vi "FGV Map Get Data (Variant).vi"(8 "error in (no error)":errorcluster, 10 "Data Key":string, 11 "Instance Key":string) -> (0 "error out":errorcluster, 2 "Data Not Found ?":bool, 3 "Data Out":variant)   [LabVIEW 2020, in "FGV Map.lvlib"]
uses:
  FGV Map.lvlib
  Controls/FGV Map Core State.ctl
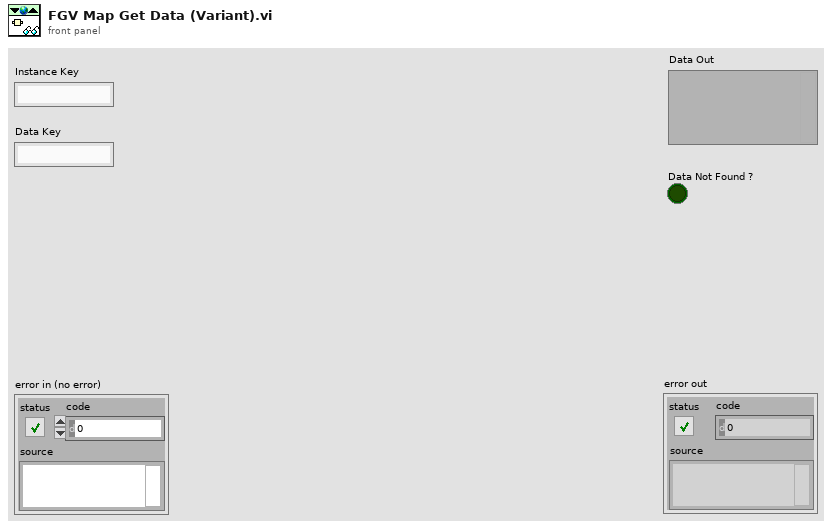
[diagram p1: front panel]
types:
  T1 = typedef "FGV Map.lvlib/FGV Map Core State.ctl" = enum16{"Init", "Set Instance (Unlock)", "Get Instance", "Get Instance (Lock)", "Unlock", "Get All Instances", "Delete Instance"}
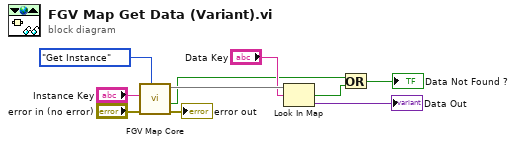
[diagram p0: block diagram]
diagram:
  n1 = call "FGV Map Core.vi"("FGV State"=FGV_Map_Core_State."Get Instance", "error in"="error in (no error)", "Instance Key"="Instance Key") -> ("error out"=→"error out":errorcluster, "Instance Not Found ?"=w4:bool, "Instance Out"=w7:map{string, variant})  [unwired: 4 in, 2 out]
  n2 = Look In Map(map=w7, key="Data Key") -> (key not found?=w3:bool, value=→"Data Out":variant)  [unwired: 1 in]
  n3 = Or(x=w4, y=w3) -> (x .or. y?=→"Data Not Found ?":bool)
